vi "ClientDemo.vi"() -> ()   [LabVIEW 2020]
uses:
  lib/SnapMB.lvlib
panel:
  out "Write":string="No Error"
  in  "Write Start":u16=17
  out "Read":string="No Error"
  in  "Scan time (ms)":u32=100
  in  "Address":string="127.0.0.1"
  in  "Proto":i32(ring) items=["TCP", "UDP", "RTUOverTCP", "RTUOverUDP"]
  in  "Port":u16=502
  out "JobTime (ms)":i32
  out "Connected":bool
  out "error out":errorcluster
  out "Run":bool
  in  "?":bool
  in  "Amount":u16=16
  in  "Read Start":u16=1
  out "RD Data":u16[](array[numeric]) format="%x"
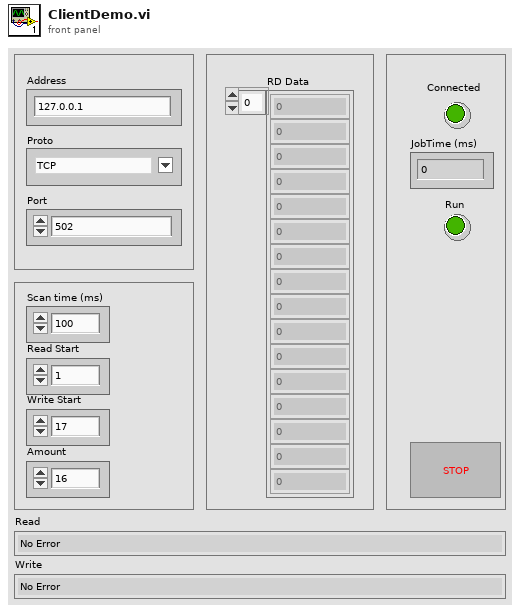
[diagram p1: front panel]
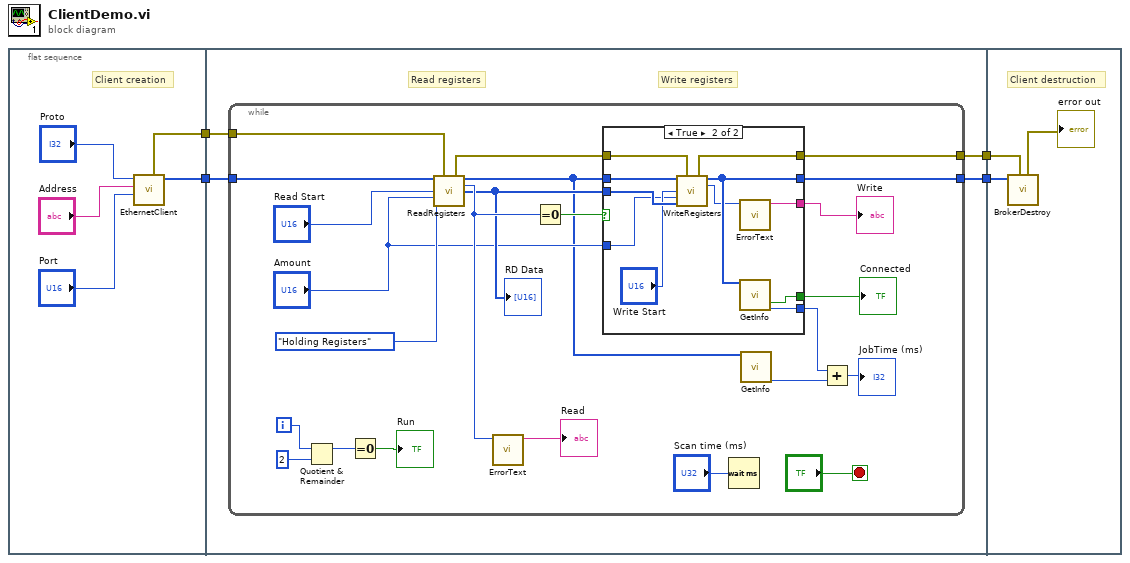
[diagram p0: block diagram]
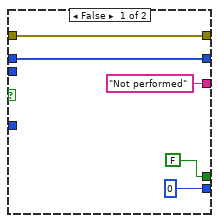
[diagram p2: hidden frame]
diagram:
  n1 = flat-sequence {
    tunnel: [w6] -> w4
    tunnel: [w5] -> w3
    tunnel: w4 -> [w13]
    tunnel: w3 -> [w12]
    tunnel: [w11] -> w2
    tunnel: [w10] -> w1
    tunnel: w2 -> [w55]
    tunnel: w1 -> [w54]
    frame #0 {
      # "Client creation"
      n2 = call "EthernetClient.vi"("Port"="Port", "Address"="Address", "Proto"="Proto") -> ("Client"=w6:u64[], "error out"=w5:errorcluster)  [unwired: 5 in]
    }
    frame #1 {
      # "Write registers"
      # "Read registers"
      n3 = while {
        tunnel: w13 -> [w32]
        tunnel: w12 -> [w31]
        tunnel: [w21] -> w11
        tunnel: [w19] -> w10
        i -> [w37]
        stop <- "?" stop-if-true
        n4 = Quotient & Remainder(x=w37, y=2) -> (x-y*floor(x/y)=w35:i32)  [unwired: 1 out]
        n5 = Equal To 0?(x=w35) -> (x = 0?=→"Run":bool)
        n6 = call "ReadRegisters.vi"("Handle In"=w32, "error in (no error)"=w31, "Read Start"="Read Start", "Read Amount"="Amount", "Area"=enum16{"Holding Registers", "Input Registers"}."Holding Registers") -> ("error out"=w20:errorcluster, "Handle Out"=w22:u64[], "Result"=w25:i32, "RD Data"=w24:u16[])  [unwired: 7 in]
        "RD Data" <- w24
        n7 = call "ErrorText.vi"("ErrNo"=w25) -> ("ErrMessage"=→"Read":string)  [unwired: 9 in, 1 out]
        n8 = Equal To 0?(x=w25) -> (x = 0?=w26:bool)
        n9 = case shown="True" w26 {
          tunnel: w22 -> [w41 w53]
          tunnel: w24 -> [_ w52]
          tunnel: "Amount" -> [_ w50]
          tunnel: [w41 w47] -> w21
          tunnel: w20 -> [w42 w49]
          tunnel: [w42 w48] -> w19
          tunnel: [0 ("JobTime") w46] -> w17
          tunnel: [FALSE ("Connected") w45] -> w15
          tunnel: ["Not performed" ("ErrMessage") w44] -> w14
          frame False {
          }
          frame True {
            n10 = call "WriteRegisters.vi"("Handle In"=w53, "error in (no error)"=w49, "Write Start"="Write Start", "Write Amount"=w50, "WR Data"=w52) -> ("error out"=w48:errorcluster, "Handle Out"=w47:u64[], "Result"=w43:i32)  [unwired: 7 in, 1 out]
            n11 = call "ErrorText.vi"("ErrNo"=w43) -> ("ErrMessage"=w44:string)  [unwired: 9 in, 1 out]
            n12 = call "GetInfo.vi"("Broker In"=w47) -> ("Connected"=w45:bool, "JobTime"=w46:i32)  [unwired: 12 in, 5 out]
          }
        }
        "Connected" <- w15
        "Write" <- w14
        n13 = Wait (ms)(milliseconds to wait="Scan time (ms)") -> ()  [unwired: 1 out]
        n14 = call "GetInfo.vi"("Broker In"=w22) -> ("JobTime"=w16:i32)  [unwired: 12 in, 6 out]
        n15 = Add(x=w17, y=w16) -> (x+y=→"JobTime (ms)":i32)
      }
    }
    frame #2 {
      # "Client destruction"
      n16 = call "BrokerDestroy.vi"("error in (no error)"=w54, "Handle In"=w55) -> ("error out"=→"error out":errorcluster)  [unwired: 9 in]
    }
  }
